vi "LHF.DB.Mongo.Collection.Remove.vi"(8 "error in (no error)":errorcluster, 9 "query":variant, 10 "collectionName":string, 11 "LHF.DB.Mongo in":refnum<class "LHF.DB.Mongo.lvclass">) -> (0 "error out":errorcluster, 3 "LHF.DB.Mongo out":refnum<class "LHF.DB.Mongo.lvclass">)   [LabVIEW 2013, in "LHF.DB.Mongo.lvclass"]
uses:
  LHF.DB.Mongo.lvclass
  C:/Users/Ricardo/Desktop/Projetos/LabVIEW-MongoDB/src/Driver/MongoDB.Driver.dll
  Driver/MongoDB.Driver.dll
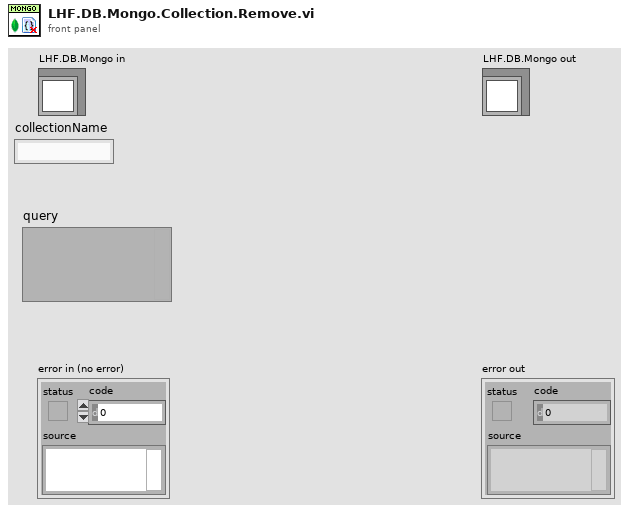
[diagram p1: front panel]
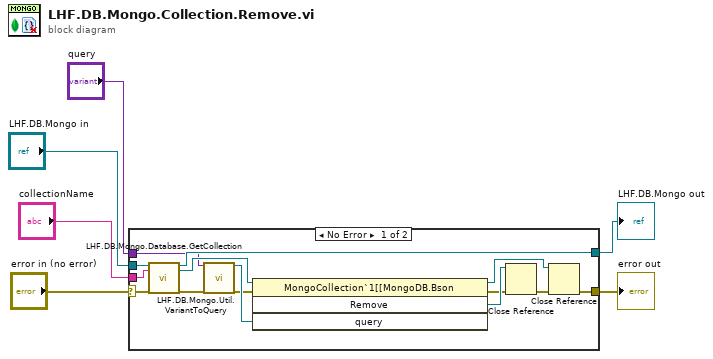
[diagram p0: block diagram]
diagram:
  n1 = case shown="No Error" "error in (no error)" {
    selector: "error in (no error)" -> [w15 w22]
    tunnel: [w18 w21] -> w4
    tunnel: "LHF.DB.Mongo in" -> [w19 w21]
    tunnel: "collectionName" -> [w20 _]
    tunnel: "query" -> [w10 _]
    tunnel: [w11 w22] -> w1
    frame No Error {
      n2 = call "LHF.DB.Mongo.Database.GetCollection.vi"("LHF.DB.Mongo in"=w19, "collectionName"=w20, "error in (no error)"=w15) -> ("LHF.DB.Mongo in"=w18:refnum<class "LHF.DB.Mongo.lvclass">, "MongoCollection"=w17:refnum<k24>, "error out"=w7:errorcluster)  [unwired: 14 in]
      n3 = call "LHF.DB.Mongo.Util.VariantToQuery.vi"("Equal"=w10, "error in (no error)"=w7) -> (".NET Refnum out"=w9:refnum<k24>, "error out"=w8:errorcluster)  [unwired: 16 in]
      n4 = invoke class="MongoCollection`1[[MongoDB.Bson" method="Remove"(reference=w17, error in=w8, "query"=w9) -> (reference out=w14:refnum<k24>, error out=w13:errorcluster, "Remove"=w16:refnum<k24>)  [unwired: 1 in, 1 out]
      n5 = Close Reference(reference=w16, error in (no error)=w13) -> (error out=w12:errorcluster)
      n6 = Close Reference(reference=w14, error in (no error)=w12) -> (error out=w11:errorcluster)
    }
    frame Error {
    }
  }
  "error out" <- w1
  "LHF.DB.Mongo out" <- w4
